vi "TP.CM BAM.vi"(5 "Source Address":u8=27, 7 "PGN":u32 format="%.0x", 9 "Total Message Size(bytes)":u16, 11 "Total Number of Packets":u8) -> (4 "Arb ID":u32 format="%.0x", 8 "Data":u8[](array[numeric]) format="%.0x")   [LabVIEW 2015, in "J1939 Addon Shared.lvlib" / "J1939 Utilities.lvlib"]
uses:
  J1939 Utilities.lvlib
  Types/PGN Fields Cluster.ctl
  Convert J1939 ID to CAN Arb ID.vi
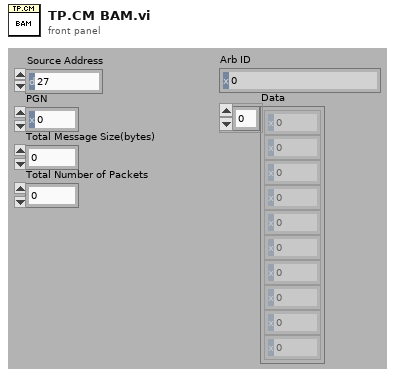
[diagram p1: front panel]
types:
  T1 = typedef "J1939 Addon Shared.lvlib/J1939 Utilities.lvlib/PGN Fields Cluster.ctl" = cluster{"Reserved Bit":u8, "Data page":u8, "PDU Format":u8, "PDU Specific":u8}
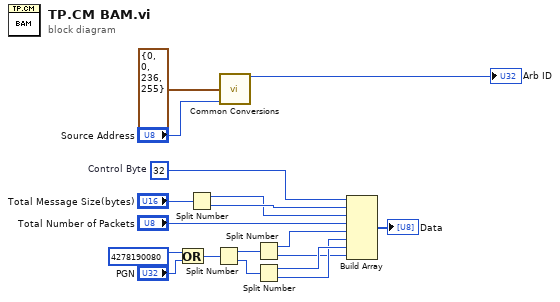
[diagram p0: block diagram]
diagram:
  w12 = u8 32  # Control Byte
  n1 = Or(x=u32 4278190080, y="PGN") -> (x .or. y?=w6:u32)
  n2 = Split Number(x="Total Message Size(bytes)") -> (hi(x)=w10:u8, lo(x)=w11:u8)
  n3 = Split Number(x=w6) -> (hi(x)=w7:u16, lo(x)=w8:u16)
  n4 = call-poly "Common Conversions.vi"("PGN Fields"=T1 {"Reserved Bit"=0, "Data page"=0, "PDU Format"=236, "PDU Specific"=255}, "Source Address"="Source Address") -> ("ID"=→"Arb ID":u32)  [unwired: 3 in, 10 out]
  n5 = Split Number(x=w7) -> (hi(x)=w5:u8, lo(x)=w1:u8)
  n6 = Split Number(x=w8) -> (hi(x)=w4:u8, lo(x)=w2:u8)
  n7 = Build Array(w12, w11, w10, "Total Number of Packets", w5, w2, w4, w1) -> (→"Data":u8[])
